vi "D4.vi"(1 "x":i64) -> (0 "64bit integer":i64)   [LabVIEW 2012]
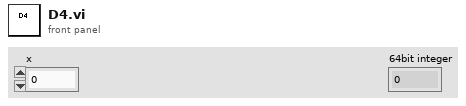
[diagram p1: front panel]
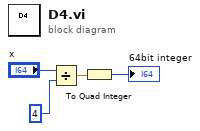
[diagram p0: block diagram]
diagram:
  n1 = Divide(x="x", y=4) -> (x/y=w3:dbl)
  n2 = To Quad Integer(1:w3) -> (0:→"64bit integer":i64)
